vi "FileParserTemp.vi"() -> ()   [LabVIEW 2017]
doc: "This is my file parser. It take a macro file as an input and reads temperature control parameters and time control parameters."
uses:
  typedefs/temp control params.ctl
  typedefs/time control params.ctl
panel:
  out "time control parameters":T1 {"Measurment time interval" format="%.2e"}
  out "temp control parameters":T2 {"End Temp" format="%.2f"; "Temp Step" format="%.2f"; "Start Temp" format="%.2f"}
  out "file path used":path
  out "Auto Launch Data Viewer at End":bool
  # "Initialization File Parser"
  # "Charles Kinzel\nPHYS 350\nAss 5"
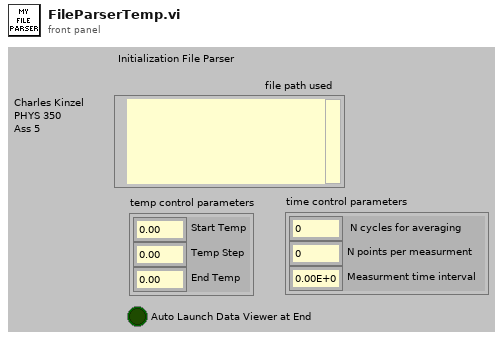
[diagram p1: front panel]
types:
  T1 = typedef "time control params.ctl" = cluster{"N cycles for averaging":i32, "N points per measurment":i32, "Measurment time interval":dbl}
  T2 = typedef "temp control params.ctl" = cluster{"Start Temp":dbl, "Temp Step":dbl, "End Temp":dbl}
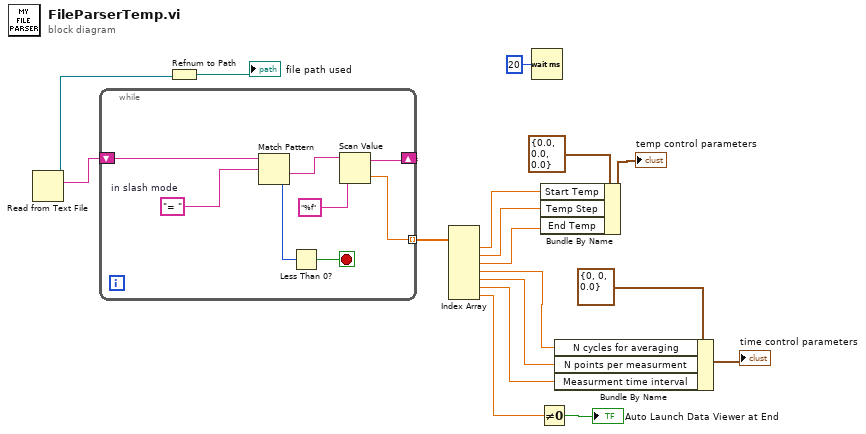
[diagram p0: block diagram]
diagram:
  n1 = Read from Text File() -> (refnum out=w2:refnum<file>, text=w15:string)  [unwired: 4 in, 2 out]
  n2 = while {
    shift-right: [w21] -> _
    shift-left: w15 -> [w24]
    tunnel: [w20] -> w14 mode=indexing
    stop <- w18 stop-if-true
    w25 = "= "  # in slash mode
    n3 = Match Pattern(string=w24, regular expression=w25) -> (after substring=w23:string, offset past match=w19:i32)  [unwired: 1 in, 2 out]
    n4 = Less Than 0?(x=w19) -> (x < 0?=w18:bool)
    n5 = Scan Value(string=w23, format string="%f") -> (output string=w21:string, value=w20:dbl)  [unwired: 1 in]
  }
  n6 = Refnum to Path(1:w2) -> (0:→"file path used":path)
  n7 = Index Array(array=w14) -> (element #1=w11:dbl, element #2=w10:dbl, element #3=w9:dbl, element #4=w7:dbl, element #5=w6:dbl, element #6=w5:dbl, element #7=w4:dbl)  [unwired: 7 in]
  n8 = Wait (ms)(milliseconds to wait=u32 20) -> ()  [unwired: 1 out]
  n9 = Not Equal To 0?(x=w4) -> (x != 0?=→"Auto Launch Data Viewer at End":bool)
  n10 = Bundle By Name(cluster=T2 {"Start Temp"=0.0, "Temp Step"=0.0, "End Temp"=0.0} ("temp control parameters"), "Start Temp"=w11, "Temp Step"=w10, "End Temp"=w9) -> (→"temp control parameters":T2)
  n11 = Bundle By Name(cluster=T1 {"N cycles for averaging"=0, "N points per measurment"=0, "Measurment time interval"=0.0} ("time control parameters"), "N cycles for averaging"=w7, "N points per measurment"=w6, "Measurment time interval"=w5) -> (→"time control parameters":T1)
